vi "ReplaceMe.vi"(0 "reference in":refnum<class "G#Interface.lvclass">, 5 "error in (no error)":errorcluster) -> (14 "reference out":refnum<class "G#Interface.lvclass">, 19 "error out":errorcluster)   [LabVIEW 2020, in "G#Interface.lvclass"]
doc: "Dummy VI that is replaced by the delegated implementing method."
uses:
  <vilib>/addons/_AddQ/G#Interface/G#Interface.lvclass
  C:/Program Files (x86)/National Instruments/LabVIEW 2020/vi.lib/addons/_AddQ/G#Object/G#Object.lvclass
  <vilib>/addons/_AddQ/G#Object/G#Object.lvclass
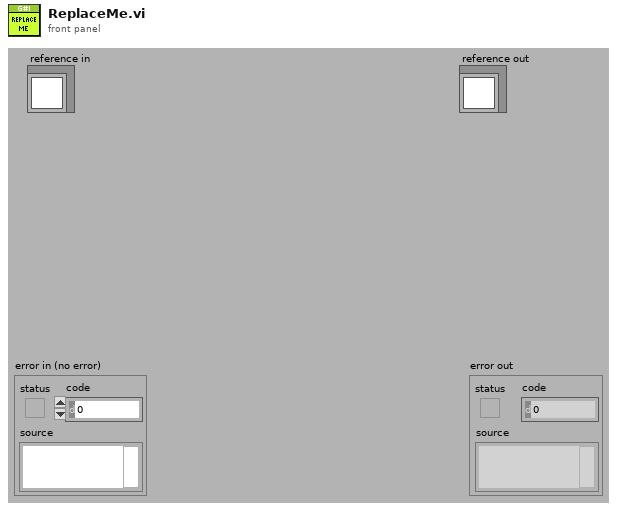
[diagram p1: front panel]
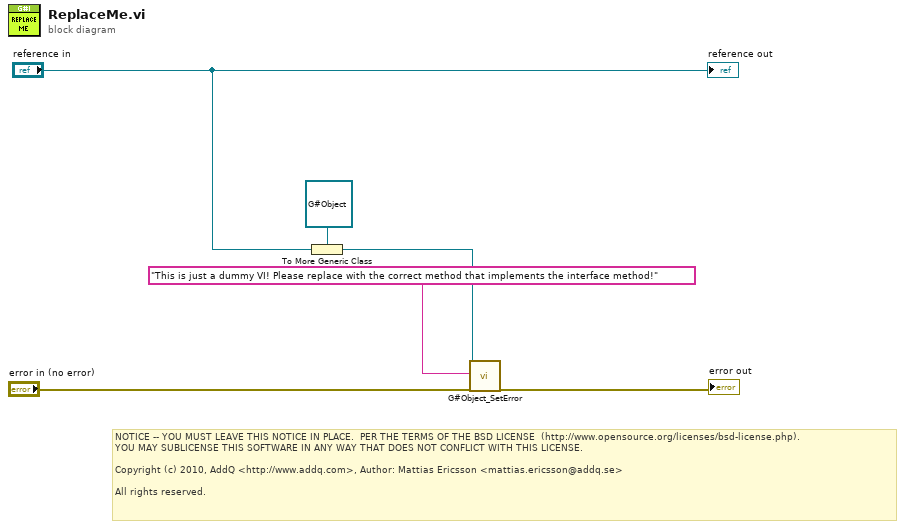
[diagram p0: block diagram]
diagram:
  # "NOTICE -- YOU MUST LEAVE THIS NOTICE IN PLACE.  PER THE TERMS OF THE BSD LICENSE  (http://www.opensource.org/licenses/bsd-license.php).\nYOU MAY SUBLICENSE THIS SOFTWARE IN ANY WAY THAT DOES NOT CONFLICT WITH THIS LICENSE.\n\nCopyright (c) 2010, AddQ <http://www.addq.com>, Author: Mattias Ericsson <mattias.ericsson@addq.se>\n\nAll rights reserved."
  n1 = To More Generic Class(target class=refnum<class "G#Object.lvclass"> refnum ("G#Object.lvclass"), reference="reference in") -> (generic class reference=w1:refnum<class "G#Object.lvclass">)
  n2 = call <vilib>:"G#Object_SetError.vi"("reference in"=w1, "source"="This is just a dummy VI! Please replace with the correct method that implements the interface method!", "error in (no error)"="error in (no error)") -> ("error out"=→"error out":errorcluster)  [unwired: 16 in]
  "reference out" <- "reference in"
